vi "GetControlType.vi"(8 "error in":errorcluster, 11 "Control in":refnum<class "Control.lvclass">) -> (0 "error out":errorcluster, 3 "Control out":refnum<class "Control.lvclass">, 4 "type string":string)   [LabVIEW 2014, in "PythonConverter_GUI.lvclass"]
uses:
  PythonConverter_GUI.lvclass
  VI Interpreter/Classes/Control/Control.lvclass
  VI Interpreter/Classes/Control/Control.lvclass/Control.ctl
  <vilib>/regexp/Match Regular Expression.xnode
  Parsing/Python Functions.lvlib
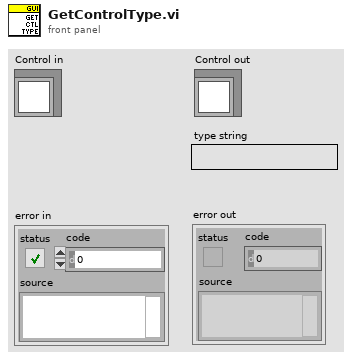
[diagram p1: front panel]
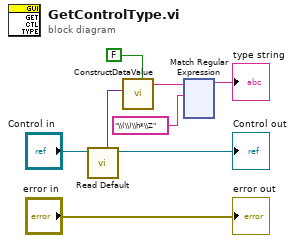
[diagram p0: block diagram]
diagram:
  n1 = call "Read Default.vi"("Control in"="Control in") -> ("Control out"=→"Control out":refnum<class "Control.lvclass">, "Default"=w3:variant)  [unwired: 7 in]
  n2 = call "ConstructDataValue.vi"("label"=FALSE, "Value"=w3) -> ("value"=w2:string)  [unwired: 6 in, 1 out]
  n3 = xnode "Match Regular Expression"("input string"=w2, "regular expression"="\\(\\)\\h*\\Z") -> ("before match"=→"type string":string)  [unwired: 4 in, 4 out]
  "error out" <- "error in"
